vi "robot_efg_server.vi"(11 "efg load":bool) -> ()   [LabVIEW 2020]
uses:
  status/stop software.vi
  status/emergency stop.vi
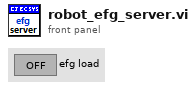
[diagram p1: front panel]
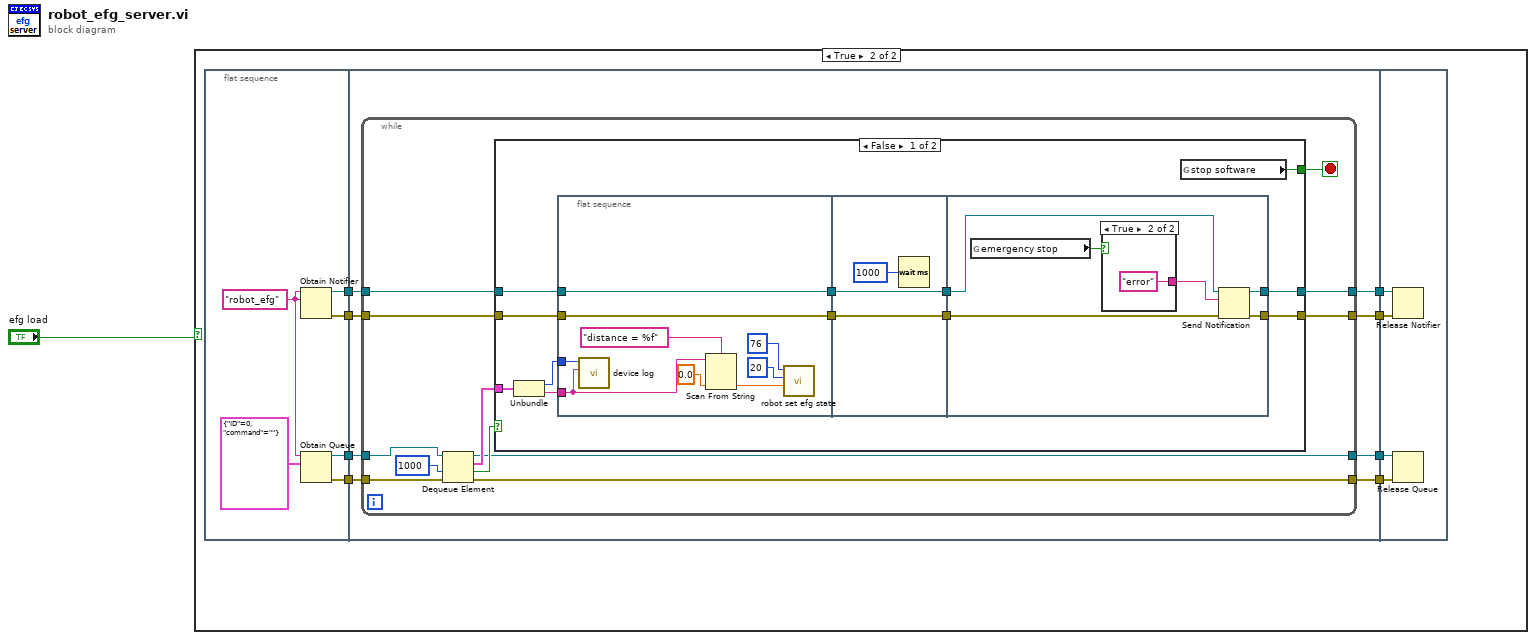
[diagram p0: block diagram]
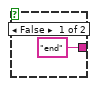
[diagram p3: hidden frame]
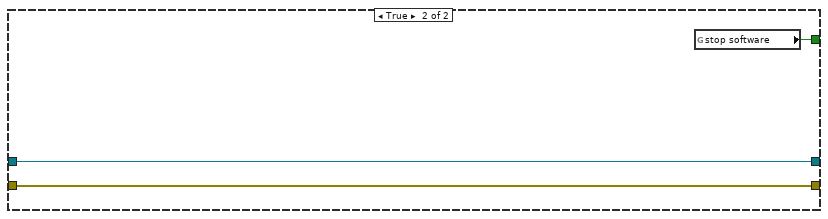
[diagram p4: hidden frame]
diagram:
  n1 = case shown="True" "efg load" {
    frame False {
    }
    frame True {
      n2 = flat-sequence {
        tunnel: [w15] -> w9
        tunnel: [w14] -> w8
        tunnel: [w13] -> w7
        tunnel: [w12] -> w6
        tunnel: w9 -> [w23]
        tunnel: w8 -> [w22]
        tunnel: w7 -> [w21]
        tunnel: w6 -> [w20]
        tunnel: [w19] -> w5
        tunnel: [w18] -> w4
        tunnel: [w17] -> w3
        tunnel: [w16] -> w2
        tunnel: w5 -> [w74]
        tunnel: w4 -> [w73]
        tunnel: w3 -> [w72]
        tunnel: w2 -> [w71]
        frame #0 {
          w11 = "robot_efg" ("name (unnamed)")
          n3 = Obtain Notifier(name (unnamed)=w11, notification data type=w11) -> (notifier out=w13:refnum<notifier>, error out=w12:errorcluster)  [unwired: 2 in, 1 out]
          n4 = Obtain Queue(name (unnamed)=w11, element data type=cluster{"ID":i32, "command":string} {"ID"=0, "command"=""} ("参数")) -> (queue out=w15:refnum<queue>, error out=w14:errorcluster)  [unwired: 3 in, 1 out]
        }
        frame #1 {
          n5 = while {
            tunnel: w23 -> [w35]
            tunnel: w22 -> [w34]
            tunnel: w21 -> [w28]
            tunnel: w20 -> [w29]
            tunnel: [w27] -> w19
            tunnel: [w26] -> w18
            tunnel: [w25] -> w17
            tunnel: [w24] -> w16
            stop <- w30 stop-if-true
            n6 = Dequeue Element(queue=w35, timeout in ms (-1)=1000, error in (no error)=w34) -> (queue out=w25:refnum<queue>, element=w31:cluster{"ID":i32, "command":string}, timed out?=w32:bool, error out=w24:errorcluster)
            n7 = case shown="False" w32 {
              tunnel: w31 -> [w38 _]
              tunnel: [w39 w68] -> w30
              tunnel: w29 -> [w47 w70]
              tunnel: w28 -> [w46 w69]
              tunnel: [w45 w69] -> w27
              tunnel: [w44 w70] -> w26
              frame False {
                n8 = Unbundle(w38) -> ("ID"=w36:i32, "command"=w37:string)
                n9 = flat-sequence {
                  tunnel: w47 -> [w56]
                  tunnel: [w56] -> w43
                  tunnel: w46 -> [w55]
                  tunnel: [w55] -> w41
                  tunnel: w37 -> [w53]
                  tunnel: w36 -> [w54]
                  tunnel: w43 -> [w59]
                  tunnel: [w59] -> w42
                  tunnel: w41 -> [w58]
                  tunnel: [w58] -> w40
                  tunnel: w42 -> [w64]
                  tunnel: w40 -> [w63]
                  tunnel: [w62] -> w45
                  tunnel: [w61] -> w44
                  frame #0 {
                    n10 = call "device log.vi"("new element/subarray"=w53, "worker ID"=w54) -> ()  [unwired: 10 in]
                    n11 = Scan From String(format string="distance = %f", input string=w53, default 1=sgl 0.0) -> (output 1=w52:sgl)  [unwired: 2 in, 3 out]
                    n12 = call "robot set efg state.vi"("distance"=w52, "type"=20, "robot_id"=76) -> ()  [unwired: 8 in, 1 out]
                  }
                  frame #1 {
                    n13 = Wait (ms)(milliseconds to wait=u32 1000) -> ()  [unwired: 1 out]
                  }
                  frame #2 {
                    n14 = global read "emergency stop.vi" "emergency stop"() -> (w60:bool)
                    n15 = case shown="True" w60 {
                      tunnel: ["end" ("notification") "error" ("notification")] -> w65
                      frame False {
                      }
                      frame True {
                      }
                    }
                    n16 = Send Notification(notification=w65, notifier=w63, error in (no error)=w64) -> (notifier out=w62:refnum<notifier>, error out=w61:errorcluster)
                  }
                }
                n17 = global read "stop software.vi" "stop software"() -> (w39:bool)
              }
              frame True {
                n18 = global read "stop software.vi" "stop software"() -> (w68:bool)
              }
            }
          }
        }
        frame #2 {
          n19 = Release Notifier(notifier=w74, error in (no error)=w73) -> ()  [unwired: 1 in, 3 out]
          n20 = Release Queue(queue=w72, error in (no error)=w71) -> ()  [unwired: 1 in, 3 out]
        }
      }
    }
  }
